vi "SRingThreadIsOFF.vi"() -> (0 "ThreadIsOFF":u8)   [LabVIEW 2014]
uses:
  ESLSCDLL.dll
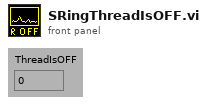
[diagram p1: front panel]
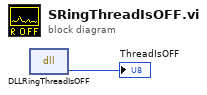
[diagram p0: block diagram]
diagram:
  n1 = dll-call lib="C:/Users/Gerhard/Documents/New64/lv/1cam/board.vis/ESLSCDLL.dll" fn="DLLRingThreadIsOFF"() -> ("Rückgabetyp"=→"ThreadIsOFF":u8)  [unwired: 3 in, 2 out]
